vi "Hood Angles LUT.vi"(10 "Hood Man Request?":bool, 11 "Shooter States":T2) -> (2 "Hood States To Dashboard":T1, 3 "Hood Angle Setpoint":dbl)   [LabVIEW 2015]
uses:
  Typedefs/Shooter States.ctl
  Typedefs/Hood States.ctl
panel:
  in  "Hood Angles LUT":dbl[](array[numeric])
  # "Hood Manual"
  # "Far"
  # "Close"
  # "Intermediate"
  # "Spy"
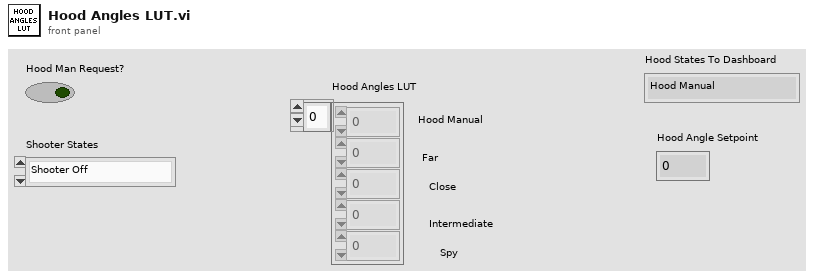
[diagram p1: front panel]
types:
  T1 = typedef "Hood States.ctl" = enum16{"Hood Manual ", "Hood Close Shot", "Hood Far Shot", "Hood Spy Shot", "Hood Intermediate"}
  T2 = typedef "Shooter States.ctl" = enum16{"Shooter Off", "Shooter Far", "Shooter Close", "Shooter Intermediate", "Shooter Spy"}
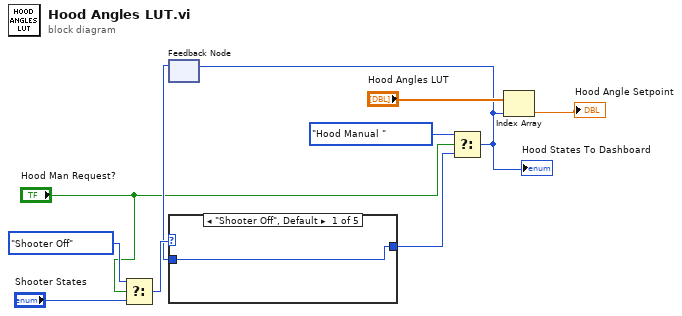
[diagram p0: block diagram]
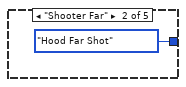
[diagram p2: hidden frame]
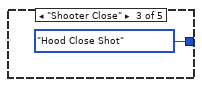
[diagram p3: hidden frame]
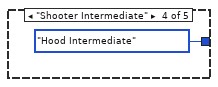
[diagram p4: hidden frame]
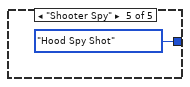
[diagram p5: hidden frame]
diagram:
  n1 = Select(t=Shooter_States."Shooter Off", s="Hood Man Request?", f="Shooter States") -> (s? t:f=w7:T2)
  n2 = feedback #1() -> (w3:T1)  [unwired: 1 in]
  n3 = case shown="\"Shooter Off\", Default" w7 {
    tunnel: [w11 Hood_States."Hood Far Shot" ("Hood States") Hood_States."Hood Close Shot" ("Hood States") Hood_States."Hood Intermediate" ("Hood States") Hood_States."Hood Spy Shot" ("Hood States")] -> w6
    tunnel: w3 -> [w11 _ _ _ _]
    frame "Shooter Off", Default {
    }
    frame "Shooter Far" {
    }
    frame "Shooter Close" {
    }
    frame "Shooter Intermediate" {
    }
    frame "Shooter Spy" {
    }
  }
  n4 = Select(t=Hood_States."Hood Manual ", s="Hood Man Request?", f=w6) -> (s? t:f=w4:T1)
  "Hood States To Dashboard" <- w4
  n5 = feedback-in #1(w4) -> ()
  n6 = Index Array(array="Hood Angles LUT", index=w4) -> (element=→"Hood Angle Setpoint":dbl)
